vi "TIFF-Write Page.vi"(0 "state in":T1={"file"=refnum, "IFD"=[], "offset"=0, "byte order"=enum."little-endian", "image size"=0, "IFD size"=0, "max frames"=0, "frames"=0}, 5 "Image Pixels (U16)":u16[][](array[numeric]), 11 "error in":errorcluster) -> (4 "state out":T1={"file"=refnum, "IFD"=[], "offset"=0, "byte order"=enum."little-endian", "image size"=0, "IFD size"=0, "max frames"=0, "frames"=0}, 15 "error out":errorcluster)   [LabVIEW 2020]
doc: "This VI writes an image array to a multipage tif file. Valid formats are U8 or U16."
uses:
  TIFF-Write State.ctl
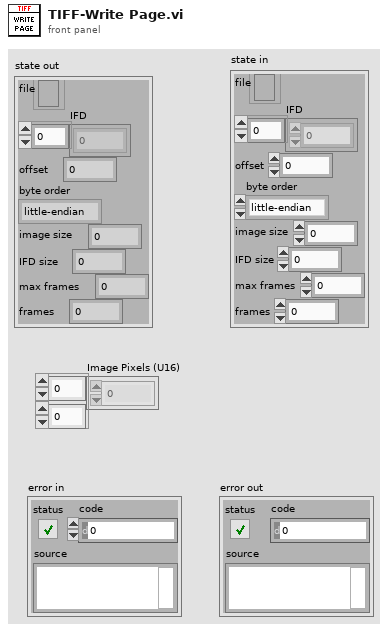
[diagram p1: front panel]
types:
  T1 = typedef "TIFF-Write State.ctl" = cluster{"file":refnum<file>, "IFD":u8[], "offset":u32, "byte order":enum16{"big-endian, network order", "native, host order", "little-endian"}, "image size":u32, "IFD size":u32, "max frames":u32, "frames":u32}
  T2 = enum16{"big-endian, network order", "native, host order", "little-endian"}
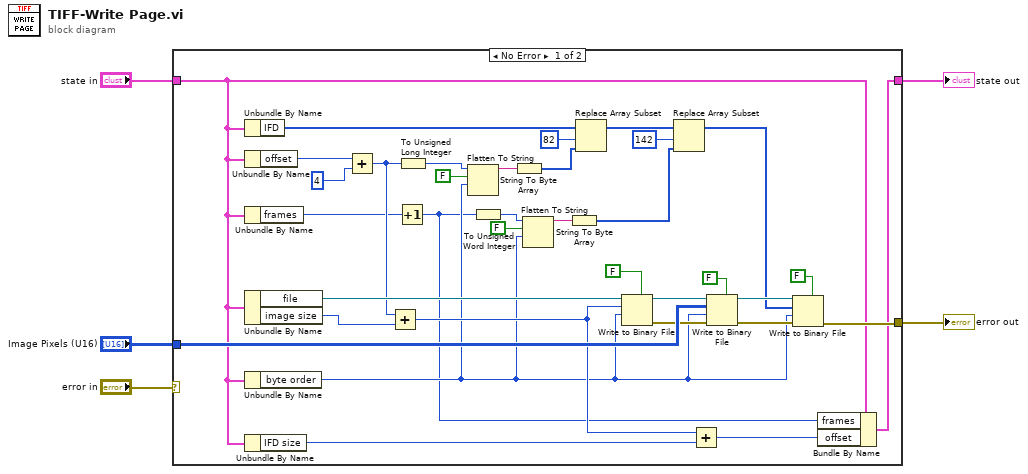
[diagram p0: block diagram]
diagram:
  n1 = case shown="No Error" "error in" {
    selector: "error in" -> [_ w42]
    tunnel: [w29 w42] -> w5
    tunnel: "Image Pixels (U16)" -> [w31 _]
    tunnel: "state in" -> [w9 w41]
    tunnel: [w18 w41] -> w1
    frame No Error {
      n2 = Unbundle By Name(w9) -> ("IFD"=w39:u8[])
      n3 = Unbundle By Name(w9) -> ("offset"=w38:u32)
      n4 = Unbundle By Name(w9) -> ("frames"=w8:u32)
      n5 = Unbundle By Name(w9) -> ("file"=w27:refnum<file>, "image size"=w24:u32)
      n6 = Unbundle By Name(w9) -> ("byte order"=w12:T2)
      n7 = Unbundle By Name(w9) -> ("IFD size"=w17:u32)
      n8 = Add(x=w38, y=u32 4) -> (x+y=w21:u32)
      n9 = Add(x=w21, y=w24) -> (x+y=w20:u32)
      n10 = Increment(x=w8) -> (x+1=w7:u32)
      n11 = To Unsigned Long Integer(number=w21) -> (unsigned 32bit integer=w34:u32)
      n12 = Flatten To String(anything=w34, prepend array or string size? (T)=FALSE, byte order (0:big-endian, network order)=w12) -> (data string=w36:string)  [unwired: 1 in, 2 out]
      n13 = To Unsigned Word Integer(number=w7) -> (unsigned 16bit integer=w6:u16)
      n14 = String To Byte Array(string=w36) -> (unsigned byte array=w35:u8[])
      n15 = Flatten To String(anything=w6, prepend array or string size? (T)=FALSE, byte order (0:big-endian, network order)=w12) -> (data string=w13:string)  [unwired: 1 in, 2 out]
      n16 = String To Byte Array(string=w13) -> (unsigned byte array=w11:u8[])
      n17 = Replace Array Subset(array=w39, new element=w35, index=82) -> (w16:u8[])
      n18 = Write to Binary File(file (use dialog)=w27, data=w20, 5:FALSE ("prepend array or string size? (T)"), 9:w12) -> (refnum out=w26:refnum<file>, error out=w25:errorcluster)  [unwired: 2 in, 1 out]
      n19 = Replace Array Subset(array=w16, new element=w11, index=142) -> (w15:u8[])
      n20 = Add(x=w20, y=w17) -> (x+y=w19:u32)
      n21 = Write to Binary File(file (use dialog)=w26, data=w31, error in=w25, 5:FALSE ("prepend array or string size? (T)"), 9:w12) -> (refnum out=w32:refnum<file>, error out=w30:errorcluster)  [unwired: 1 in, 1 out]
      n22 = Write to Binary File(file (use dialog)=w32, data=w15, error in=w30, 5:FALSE ("prepend array or string size? (T)"), 9:w12) -> (error out=w29:errorcluster)  [unwired: 1 in, 2 out]
      n23 = Bundle By Name(cluster=w9, "frames"=w7, "offset"=w19) -> (w18:T1)
    }
    frame Error {
    }
  }
  "error out" <- w5
  "state out" <- w1
